vi "Stop Config.vi"(8 "error in":errorcluster, 11 "cPAS in":refnum<class "cPAS.lvclass">) -> (0 "error out":errorcluster, 3 "cPAS out":refnum<class "cPAS.lvclass">)   [LabVIEW 2014, in "cPAS.lvclass"]
doc: "Complete the configuration of the PAS. The default does nothing. It is a place holder for tasks such as closing a config file or completing any other processes not covered by the generic methods."
uses:
  cPAS.lvclass
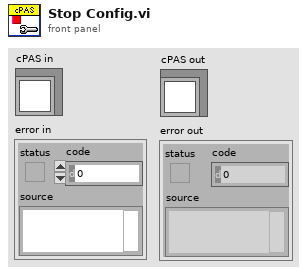
[diagram p1: front panel]
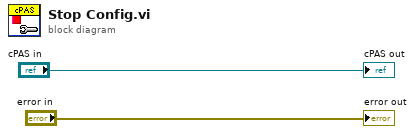
[diagram p0: block diagram]
diagram:
  "error out" <- "error in"
  "cPAS out" <- "cPAS in"
